vi "方法-循环显示.vi"(8 "error in (no error)":errorcluster caption="错误输入（无错误）", 11 "抽取参数 输入":refnum<class "抽取参数.lvclass">) -> (0 "error out":errorcluster caption="错误输出", 2 "循环显示元素":string, 3 "抽取参数 输出":refnum<class "抽取参数.lvclass">)   [LabVIEW 2020, in "抽取参数.lvclass"]
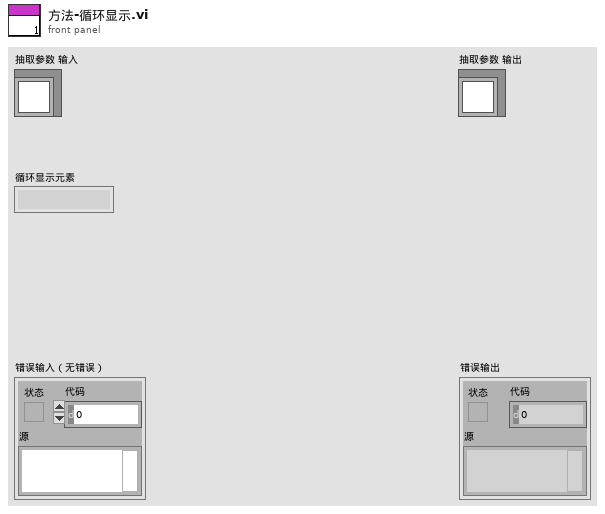
[diagram p1: front panel]
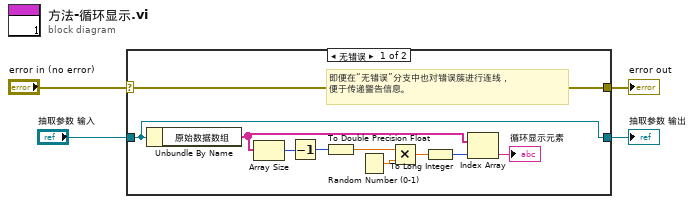
[diagram p0: block diagram]
diagram:
  n1 = case shown="无错误" "error in (no error)" {
    selector: "error in (no error)" -> [w14 w16]
    tunnel: [w14 w16] -> w3
    tunnel: [w13 w15] -> w1
    tunnel: "抽取参数 输入" -> [w13 w15]
    frame No Error {
      # "即便在“无错误”分支中也对错误簇进行连线，\n便于传递警告信息。"
      n2 = Unbundle By Name(w13) -> ("原始数据数组"=w6:string[])
      n3 = Array Size(array=w6) -> (size(s)=w12:i32)
      n4 = Decrement(x=w12) -> (x-1=w9:i32)
      n5 = To Double Precision Float(number=w9) -> (double precision float=w8:dbl)
      n6 = Random Number (0-1)() -> (number: 0 to 1=w11:dbl)
      n7 = Multiply(x=w8, y=w11) -> (x*y=w10:dbl)
      n8 = To Long Integer(number=w10) -> (32bit integer=w7:i32)
      n9 = Index Array(array=w6, index=w7) -> (element=→"循环显示元素":string)
    }
    frame Error {
    }
  }
  "error out" <- w3
  "抽取参数 输出" <- w1
